vi "sync and trig.vi"(8 "error in (no error)":errorcluster, 11 "5785_3.2GHz_one channel in":refnum<class "5785_3.2GHz_one channel.lvclass">) -> (0 "error out":errorcluster, 3 "5785_3.2GHz_one channel out":refnum<class "5785_3.2GHz_one channel.lvclass">)   [LabVIEW 2021, in "5785_3.2GHz_one channel.lvclass"]
uses:
  5785_3.2GHz_one channel.lvclass
  5785_3.2GHz_one channel.lvclass/5785_3.2GHz_one channel.ctl
  <instrlib>/_niInstr/Streaming/v1/Host/niInstr Streaming v1 Host.lvlib
  <vilib>/rvi/interface/nirviReadWriteControl/nirviReadWriteControl.xnode
  <resource>/objmgr/sessionReference.rc
  <instrlib>/_niInstr/Streaming/v1/Host/Public/Start Continuous Stream.vi
  NiFpgaLv.dll
  <vilib>/Utility/error.llb/Error Cluster From Error Code.vi
  <vilib>/rvi/interface/Simulation/niFpgaSimulationCallBeginRW.vi
  <vilib>/rvi/errors/niLvFpgaAdjustHostInterfaceError.vi
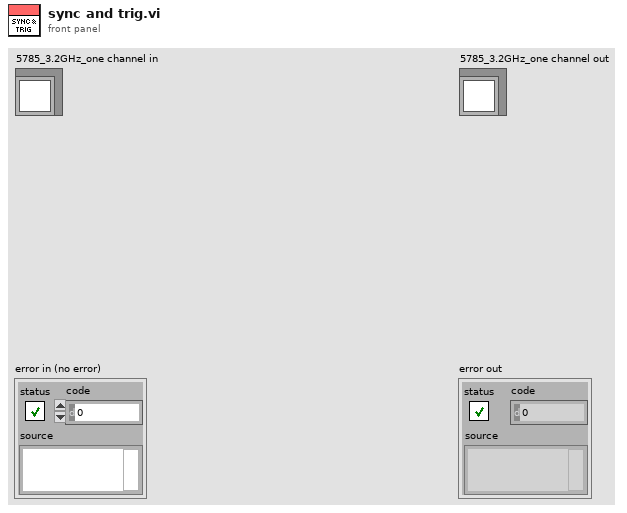
[diagram p1: front panel]
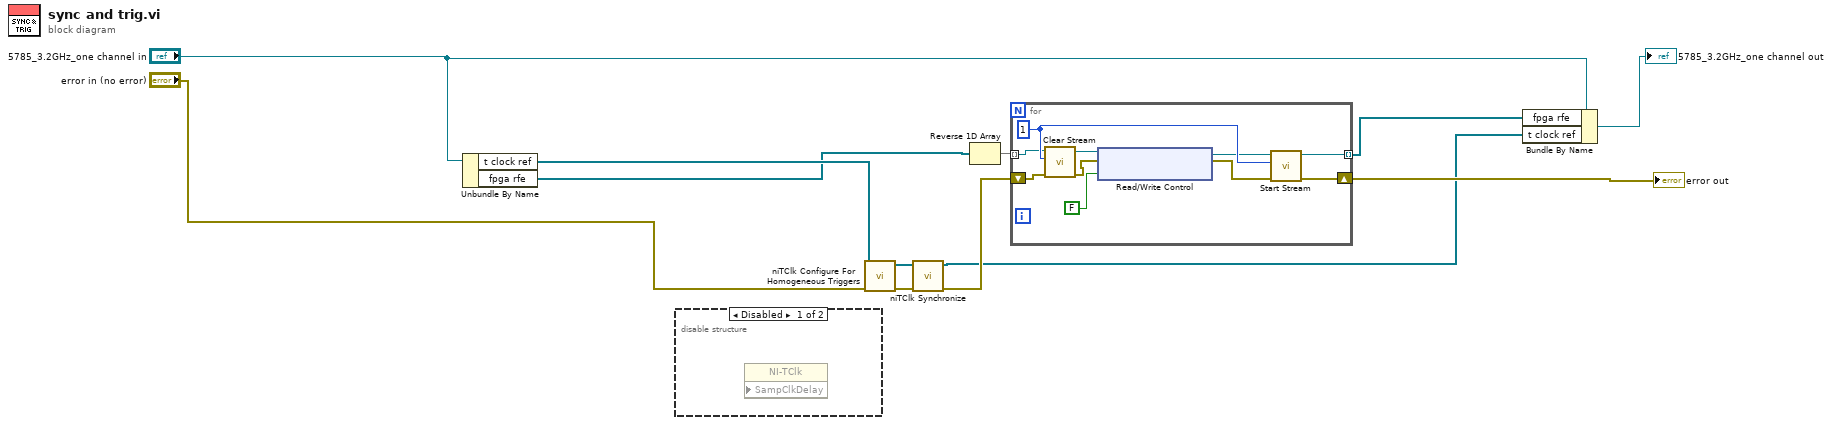
[diagram p0: block diagram]
diagram:
  n1 = Unbundle By Name("5785_3.2GHz_one channel in") -> ("t clock ref"=w8:refnum<k20>[], "fpga rfe"=w7:refnum<k20>[])
  n2 = disable-structure shown="Disabled" {
    frame Disabled {
      n3 = property class="NI-TClk" props=["SampClkDelay"]() -> ()  [unwired: 3 in, 2 out]
    }
    frame Enabled {
    }
  }
  n4 = call <instrlib>:"niTClk Configure For Homogeneous Triggers.vi"("error in (no error)"="error in (no error)", "sessions"=w8) -> ("error out"=w9:errorcluster, "sessions out"=w10:refnum<k20>[])  [unwired: 8 in]
  n5 = call <instrlib>:"niTClk Synchronize.vi"("error in (no error)"=w9, "sessions"=w10) -> ("error out"=w12:errorcluster, "sessions out"=w2:refnum<k20>[])  [unwired: 8 in]
  n6 = Reverse 1D Array(array=w7) -> (reversed array=w11:refnum<k20>[])
  n7 = for {
    tunnel: w11 -> [w18] mode=indexing
    shift-right: [w21] -> w5
    shift-left: w12 -> [w17]
    tunnel: [w20] -> w3 mode=indexing
    w22 = 1 ("stream index")
    n8 = call <instrlib>:"Clear Stream.vi"("error in (no error)"=w17, "stream index"=w22, "refnum in"=w18) -> ("error out"=w16:errorcluster, "refnum out"=w15:refnum<k20>)  [unwired: 7 in]
    n9 = xnode "Read/Write Control"("FPGA VI Reference In"=w15, "error in"=w16, "reset system clock"=FALSE) -> ("FPGA VI Reference Out"=w13:refnum<k20>, "error out"=w14:errorcluster)
    n10 = call-poly <instrlib>:"Start Stream.vi"("error in (no error)"=w14, "stream index"=w22, "refnum in"=w13) -> ("error out"=w21:errorcluster, "refnum out"=w20:refnum<k20>)  [unwired: 7 in]
  }
  "error out" <- w5
  n11 = Bundle By Name(cluster="5785_3.2GHz_one channel in", "fpga rfe"=w3, "t clock ref"=w2) -> (→"5785_3.2GHz_one channel out":refnum<class "5785_3.2GHz_one channel.lvclass">)
